vi "COB receive.vi"(6 "error in (no error)":errorcluster, 9 "Handle in":i32) -> (0 "error out":errorcluster, 1 "No data?":bool, 2 "COB id":i32, 3 "Handle out":i32, 4 "Data":u8[](array[numeric]))   [LabVIEW 2023, in "canopen.lvlib" / "CANopen.lvclass"]
doc: "Returns the oldest COB present in the reception queue."
uses:
  CANopen.lvclass
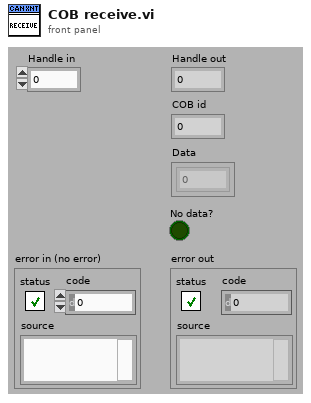
[diagram p1: front panel]
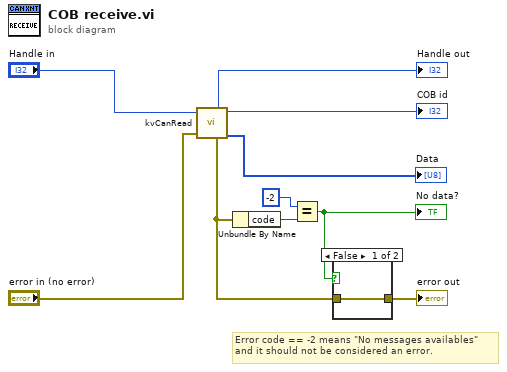
[diagram p0: block diagram]
diagram:
  # "Error code == -2 means \"No messages availables\"\nand it should not be considered an error."
  n1 = call <userlib>:"kvCanRead.vi"("error in (no error)"="error in (no error)", "Channel Handle (input only)"="Handle in") -> ("Message Data"=→"Data":u8[], "error out"=w3:errorcluster, "Channel Handle (output only)"=→"Handle out":i32, "Message Id"=→"COB id":i32)  [unwired: 1 in, 2 out]
  n2 = Unbundle By Name(w3) -> ("code"=w5:i32)
  n3 = Equal?(x=-2, y=w5) -> (x = y?=w2:bool)
  "No data?" <- w2
  n4 = case shown="False" w2 {
    tunnel: w3 -> [w11 _]
    tunnel: [w11 _] -> w1
    frame False {
    }
    frame True {
    }
  }
  "error out" <- w1
